vi "YAML Get Field Value CSV.vi"(10 "field name":string, 11 "array of strings":string[][](array[string])) -> (2 "Field Value":string)   [LabVIEW 2011]
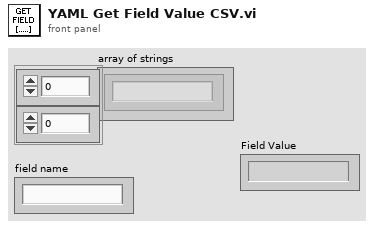
[diagram p1: front panel]
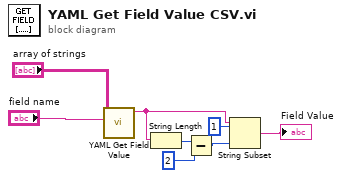
[diagram p0: block diagram]
diagram:
  n1 = call "YAML Get Field Value.vi"("field name"="field name", "array of strings"="array of strings") -> ("field value"=w2:string)  [unwired: 9 in]
  n2 = String Length(string=w2) -> (length=w6:i32)
  n3 = Subtract(x=w6, y=2) -> (x-y=w4:i32)
  n4 = String Subset(string=w2, offset (0)=1, length (rest)=w4) -> (substring=→"Field Value":string)
